vi "Untitled 8.vi"() -> ()   [LabVIEW 2013]
uses:
  Get Object Items by Path.vi
  String Subset.vi
  support/Strip Quotes and Unescape.vi
  Find Object Items by Path.vi
  support/Unescape JSON string.vi
  JSONtext.lvlib
panel:
  out "x":string
  out "op":string
  in  "<JSON>":string="{\n    \"op\": \"utx\",\n    \"x\": {\n        \"lock_time\": 0,\n        \"ver\": 1,\n        \"size\": 192,\n        \"inputs\": [\n            {\n                \"sequence\": 4294967295,\n                \"prev_out\": {\n                    \"spent\": true,\n                    \"tx_index\": 99005468,\n                    \"type\": 0,\n                    \"addr\": \"1BwGf3z7n2fHk6NoVJNkV32qwyAYsMhkWf\",\n                    \"value\": 65574000,\n                    \"n\": 0,\n                    \"script\": \"76a91477f4c9ee75e449a74c21a4decfb50519cbc245b388ac\"\n                },\n                \"script\": \"483045022100e4ff962c292705f051c2c2fc519fa775a4d8955bce1a3e29884b2785277999ed02200b537ebd22a9f25fbbbcc9113c69c1389400703ef2017d80959ef0f1d685756c012102618e08e0c8fd4c5fe539184a30fe35a2f5fccf7ad62054cad29360d871f8187d\"\n            }\n        ],\n        \"time\": 1440086763,\n        \"tx_index\": 99006637,\n        \"vin_sz\": 1,\n        \"hash\": \"0857b9de1884eec314ecf67c040a2657b8e083e1f95e31d0b5ba3d328841fc7f\",\n        \"vout_sz\": 1,\n        \"relayed_by\": \"127.0.0.1\",\n        \"out\": [\n            {\n                \"spent\": false,\n                \"tx_index\": 99006637,\n                \"type\": 0,\n                \"addr\": \"1A828tTnkVFJfSvLCqF42ohZ51ksS3jJgX\",\n                \"value\": 65564000,\n                \"n\": 0,\n                \"script\": \"76a914640cfdf7b79d94d1c980133e3587bd6053f091f388ac\"\n            }\n        ]\n    }\n}"
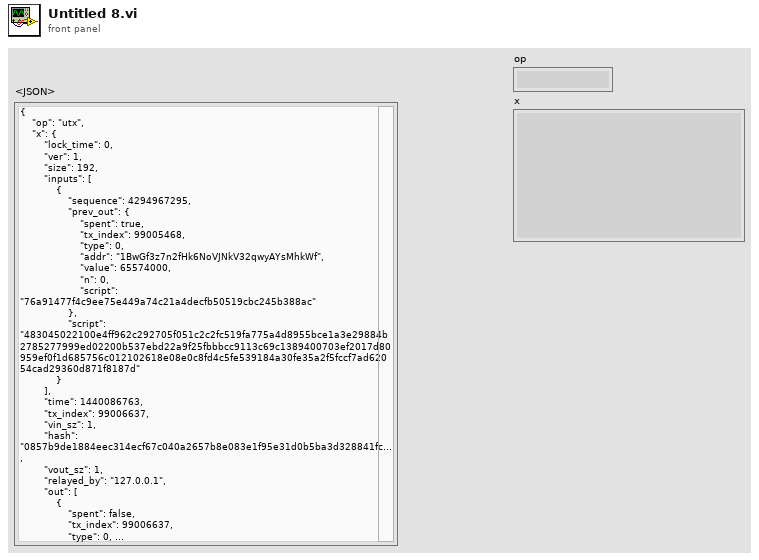
[diagram p1: front panel]
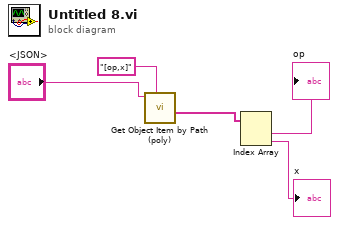
[diagram p0: block diagram]
diagram:
  n1 = call-poly "Get Object Item by Path (poly).vi"("Item Path"="[op,x]", "JSON"="<JSON>") -> ("<JSON>"=w3:string[])  [unwired: 7 in, 2 out]
  n2 = Index Array(array=w3) -> (element #1=→"op":string, element #2=→"x":string)  [unwired: 2 in]
